vi "Unflatten String To Message.vi"(0 "message string":string, 11 "error in":errorcluster) -> (4 "message":T1, 15 "error out":errorcluster)   [LabVIEW 2012, in "TLB` Template.lvlib" / "AMC.lvlib"]
uses:
  AMC.lvlib
  Message.ctl
  Tools/Keyed Array/KeyedArray.ctl
  Tools/Keyed Array/Tools_KeyedArray.lvlib
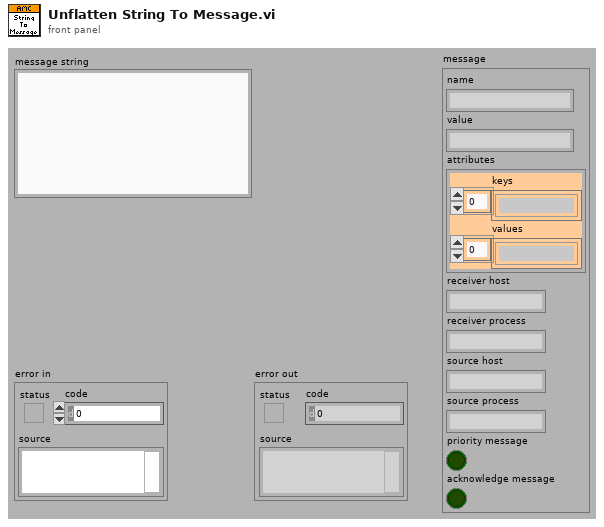
[diagram p1: front panel]
types:
  T1 = typedef "TLB` Template.lvlib/AMC.lvlib/Message.ctl" = cluster{"name":string, "value":string, "attributes":T2, "receiver host":string, "receiver process":string, "source host":string, "source process":string, "priority message":bool, "acknowledge message":bool}
  T2 = typedef "TLB` Template.lvlib/Tools_KeyedArray.lvlib/KeyedArray.ctl" = cluster{"keys":string[], "values":string[]}
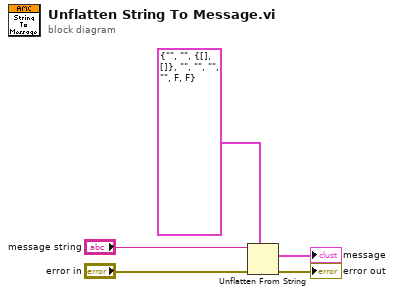
[diagram p0: block diagram]
diagram:
  n1 = Unflatten From String(type=T1 {"name"="", "value"="", "attributes"={"keys"=[], "values"=[]}, "receiver host"="", "receiver process"="", "source host"="", "source process"="", "priority message"=FALSE, "acknowledge message"=FALSE} ("message"), binary string="message string", error in (no error)="error in") -> (value=→"message":T1, error out=→"error out":errorcluster)  [unwired: 2 in, 1 out]
